vi "Set State.vi"(8 "error in (no error)":errorcluster, 10 "State":T1, 11 "Panel in":refnum<class "Panel.lvclass">) -> (0 "error out":errorcluster, 3 "Panel out":refnum<class "Panel.lvclass">)   [LabVIEW 2014, in "OOPanel.lvlib" / "Panel.lvclass"]
uses:
  Panel.lvclass
  Visibility State.ctl
  Visbility Event Data.ctl
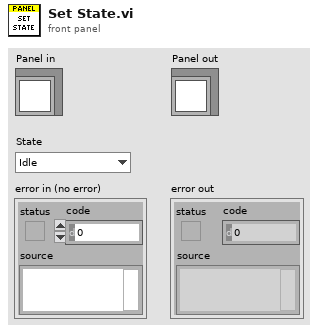
[diagram p1: front panel]
types:
  T1 = typedef "OOPanel.lvlib/Panel.lvclass/Visibility State.ctl" = enum16{"Idle", "Closed", "Hidden", "Visible", "Subpanel"}
  T2 = typedef "OOPanel.lvlib/Panel.lvclass/Visbility Event Data.ctl" = cluster{"State":T1}
  T3 = typedef "OOPanel.lvlib/Panel.lvclass/Ref Data.ctl" = cluster{"Panel Events":T4, "Panel Ref":refnum<vi>, "SubPanel":refnum<vi>, "Close":bool, "Running":bool, "State":T1}
  T4 = typedef "OOPanel.lvlib/Panel.lvclass/Panel Events.ctl" = cluster{"Visbility":refnum<user-event>, "Close":refnum<user-event>}
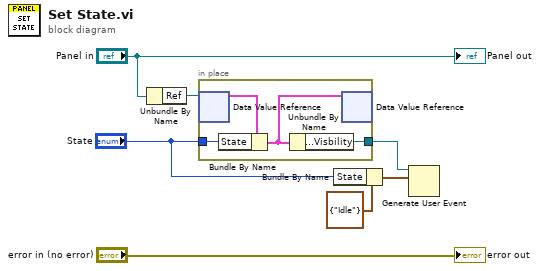
[diagram p0: block diagram]
diagram:
  n1 = Unbundle By Name("Panel in") -> ("Ref"=w6:refnum<data-value>)
  n2 = in-place {
    in-place-border: "State" -> [w10]
    in-place-border: [w8] -> w4
    n3 = in-place-dvr #1(w6) -> (w11:T3)  [unwired: 1 out]
    n4 = Bundle By Name(cluster=w11, "State"=w10) -> (w9:T3)
    n5 = Unbundle By Name(w9) -> ("Panel Events.Visbility"=w8:refnum<user-event>)
    n6 = in-place-dvr #1(w9) -> ()  [unwired: 2 out]
  }
  n7 = Bundle By Name(cluster=T2 {"State"=enum."Idle"} ("event data"), "State"="State") -> (w2:T2)
  n8 = Generate User Event(user event=w4, event data cluster=w2) -> ()  [unwired: 2 in, 2 out]
  "error out" <- "error in (no error)"
  "Panel out" <- "Panel in"
